vi "fetch_command.vi"(7 "execute command?":bool, 8 "error in (no error)":errorcluster, 11 "GenericToplevelComponent in":refnum<class "GenericToplevelComponent.lvclass">) -> (0 "error out":errorcluster, 3 "GenericToplevelComponent out":refnum<class "GenericToplevelComponent.lvclass">)   [LabVIEW 2010, in "GenericToplevelComponent.lvclass"]
uses:
  GenericToplevelComponent.lvclass
  components/Command/GenericCommand/GenericCommand/GenericCommand.lvclass
panel:
  out "command":refnum<class "GenericCommand.lvclass">
  out "# elements still in queue":i32
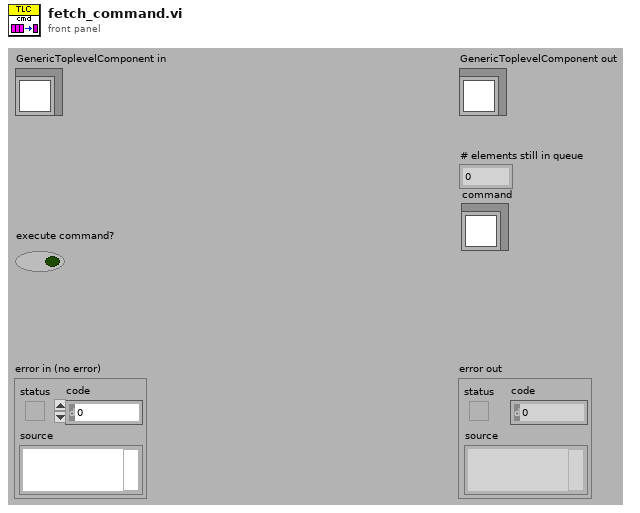
[diagram p1: front panel]
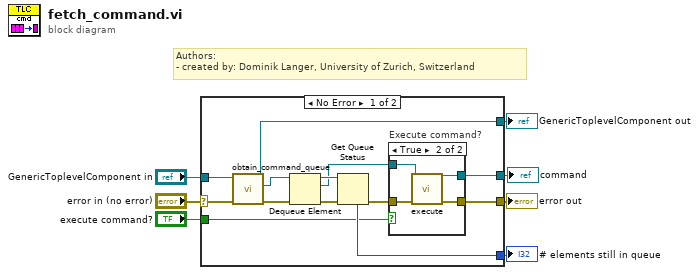
[diagram p0: block diagram]
diagram:
  # "Authors: \n- created by: Dominik Langer, University of Zurich, Switzerland"
  n1 = case shown="No Error" "error in (no error)" {
    selector: "error in (no error)" -> [w18 w28]
    tunnel: [w11 w28] -> w6
    tunnel: [w16 w27] -> w4
    tunnel: "GenericToplevelComponent in" -> [w17 w27]
    tunnel: [w13 _] -> w3
    tunnel: [w9 _] -> w2
    tunnel: "execute command?" -> [w8 _]
    frame No Error {
      n2 = call-dynamic "obtain_command_queue.vi"("error in (no error)"=w18, "GenericToplevelComponent in"=w17) -> ("error out"=w20:errorcluster, "command queue"=w15:refnum<queue>, "GenericToplevelComponent out"=w16:refnum<class "GenericToplevelComponent.lvclass">)  [unwired: 7 in]
      n3 = Dequeue Element(queue=w15, error in (no error)=w20) -> (queue out=w14:refnum<queue>, element=w10:refnum<class "GenericCommand.lvclass">, error out=w19:errorcluster)  [unwired: 1 in, 1 out]
      n4 = Get Queue Status(queue=w14, error in (no error)=w19) -> (error out=w12:errorcluster, # elements in queue=w13:i32)  [unwired: 1 in, 6 out]
      n5 = case "Execute command?" shown="True" w8 {
        tunnel: w12 -> [w22 w26]
        tunnel: [w22 w25] -> w11
        tunnel: w10 -> [w21 w24]
        tunnel: [w21 w23] -> w9
        frame False {
        }
        frame True {
          n6 = call-dynamic "execute.vi"("error in (no error)"=w26, "GenericCommand in"=w24) -> ("error out"=w25:errorcluster, "GenericCommand out"=w23:refnum<class "GenericCommand.lvclass">)  [unwired: 8 in]
        }
      }
    }
    frame Error {
    }
  }
  "error out" <- w6
  "GenericToplevelComponent out" <- w4
  "# elements still in queue" <- w3
  "command" <- w2
